vi "Tab Control Password 2012 NIVerified.vi"() -> ()   [LabVIEW 2020]
doc: "This is an example of how to password protect a tab control, which would be useful if an administrator wanted to restrict access to particular controls."
panel:
  in  "User (user)":string
  in  "OK Button":bool
  in  "Password (password)":string
  in  "stop":bool
  in  "Tab Control":T1(tab)
  out "User Name":string
  # "Overview: This is an example of how to password protect a tab control, which would be useful if an administrator wanted \nto restrict access to particular controls. \nRequirements: LabVIEW 2012 (or compatible)\nInstructions:\n1. Run the VI.\n2. Input the correct Password and User(the initial values are password and user, can be changed in Block Diagram) and click Enter.\n3. If the password and user are correct, the Password Protected Tab page will be enabled and display the user.\n4. If the password and/or user is incorrect, it will pop up a prompt dialog and stop the VI."
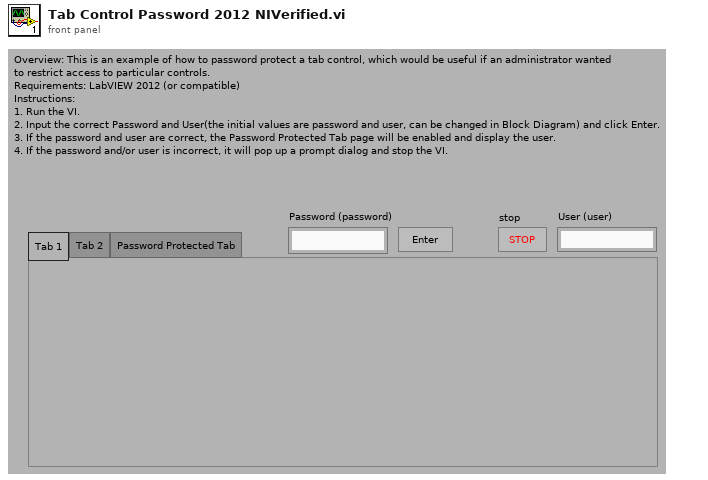
[diagram p1: front panel]
types:
  T1 = enum32{"Tab 1", "Tab 2", "Password Protected Tab"}
  T2 = enum32{"Page Enabled", "Page Disabled", "Page Disabled & Grayed"}
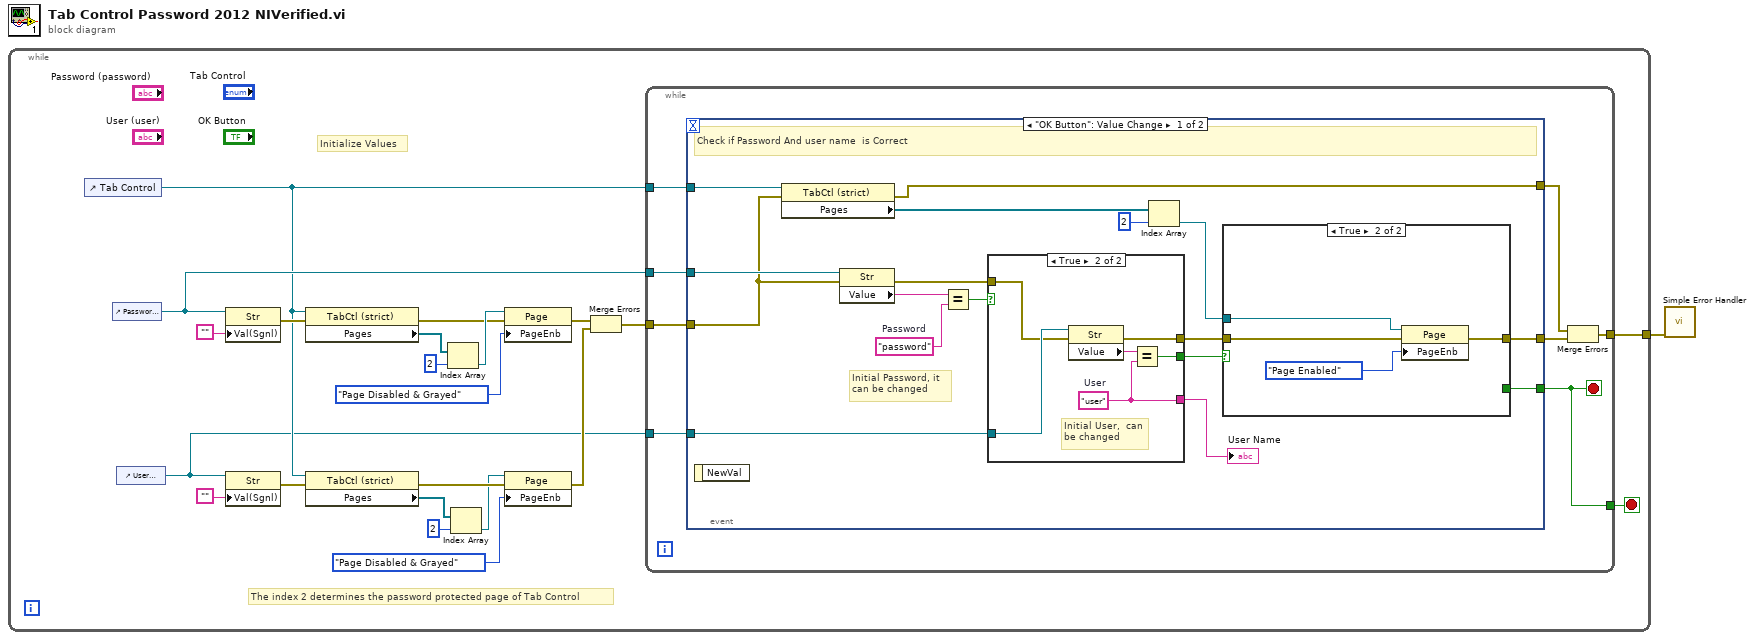
[diagram p0: block diagram]
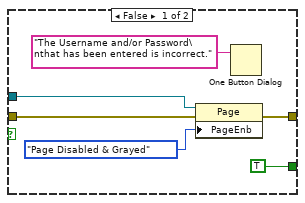
[diagram p2: hidden frame]
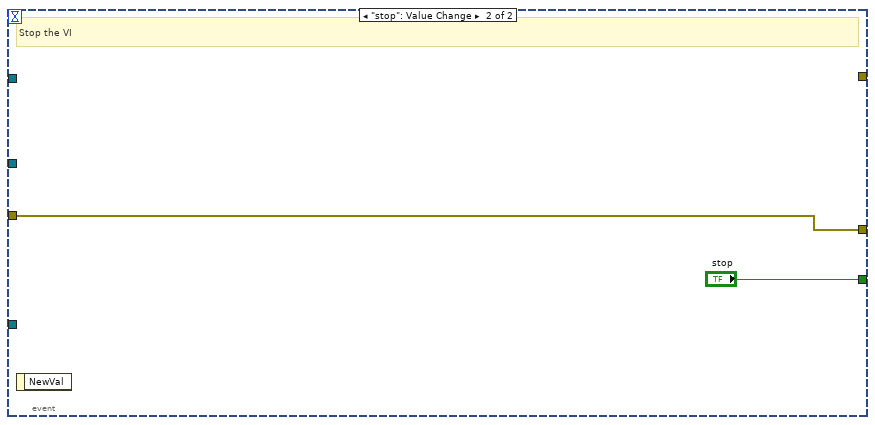
[diagram p4: hidden frame]
diagram:
  n1 = while {
    tunnel: [w2] -> w1
    stop <- w3 stop-if-true
    # "The index 2 determines the password protected page of Tab Control"
    # "Initialize Values"
    n2 = control-ref of="Tab Control"() -> (w5:refnum<vi>)
    n3 = control-ref of="Password (password)"() -> (w16:refnum<vi>)
    n4 = control-ref of="User (user)"() -> (w4:refnum<vi>)
    n5 = property on="Property Node" class="Str"(reference=w16, "Val(Sgnl)"="" ("Value (Signaling)")) -> (error out=w18:errorcluster)  [unwired: 1 in, 1 out]
    n6 = property on="Property Node" class="Str"(reference=w4, "Val(Sgnl)"="" ("Value (Signaling)")) -> (error out=w14:errorcluster)  [unwired: 1 in, 1 out]
    n7 = property on="Property Node" class="TabCtl (strict)"(reference=w5, error in=w18) -> (error out=w17:errorcluster, "Pages"=w20:refnum<vi>[])  [unwired: 1 out]
    n8 = property on="Property Node" class="TabCtl (strict)"(reference=w5, error in=w14) -> (error out=w13:errorcluster, "Pages"=w15:refnum<vi>[])  [unwired: 1 out]
    n9 = Index Array(array=w20, index=2) -> (element=w21:refnum<vi>)
    n10 = Index Array(array=w15, index=2) -> (element=w7:refnum<vi>)
    n11 = property on="Property Node" class="Page"(reference=w21, error in=w17, "PageEnb"=T2."Page Disabled & Grayed" ("Page Enabled State")) -> (error out=w9:errorcluster)  [unwired: 1 out]
    n12 = property on="Property Node" class="Page"(reference=w7, error in=w13, "PageEnb"=T2."Page Disabled & Grayed" ("Page Enabled State")) -> (error out=w10:errorcluster)  [unwired: 1 out]
    n13 = Merge Errors(w9, w10) -> (w8:errorcluster)
    n14 = while {
      tunnel: w5 -> [w31]
      tunnel: w8 -> [w30]
      tunnel: w16 -> [w29]
      tunnel: w4 -> [w28]
      tunnel: [w27] -> w3
      tunnel: [w24] -> w2
      stop <- w27 stop-if-true
      n15 = event shown="[0] \"OK Button\": Value Change" {
        selector: _ -> [_ _]
        dyn-events: _ -> [_ _]
        timeout: _ -> [_ _]
        tunnel: [w37 "stop"] -> w27
        tunnel: w31 -> [w45 _]
        tunnel: w30 -> [w36 w67]
        tunnel: w29 -> [w44 _]
        tunnel: w28 -> [w41 _]
        tunnel: [w33 w67] -> w25
        tunnel: [w32 _] -> w26
        event "OK Button": Value Change {
          w48 = "password"  # Password
          # "Initial Password, it \ncan be changed"
          # "Check if Password And user name  is Correct"
          n16 = event-data() -> ()  [unwired: 1 in, 1 out]
          n17 = property on="Property Node" class="TabCtl (strict)"(reference=w45, error in=w36) -> (error out=w32:errorcluster, "Pages"=w47:refnum<vi>[])  [unwired: 1 out]
          n18 = property on="Property Node" class="Str"(reference=w44, error in=w36) -> (error out=w35:errorcluster, "Value"=w43:string)  [unwired: 1 out]
          n19 = Equal?(x=w43, y=w48) -> (x = y?=w42:bool)
          n20 = case shown="True" w42 {
            selector: w42 -> [w60 _]
            tunnel: [w60 w65] -> w40
            tunnel: w41 -> [_ w64]
            tunnel: [_ w63] -> w38
            tunnel: w35 -> [w59 w62]
            tunnel: [w59 w61] -> w34
            frame False {
            }
            frame True {
              w63 = "user"  # User
              # "Initial User,  can\nbe changed"
              n21 = property on="Property Node" class="Str"(reference=w64, error in=w62) -> (error out=w61:errorcluster, "Value"=w66:string)  [unwired: 1 out]
              n22 = Equal?(x=w66, y=w63) -> (x = y?=w65:bool)
            }
          }
          "User Name" <- w38
          n23 = Index Array(array=w47, index=2) -> (element=w39:refnum<vi>)
          n24 = case shown="True" w40 {
            tunnel: w39 -> [w52 w57]
            tunnel: [TRUE ("stop") _] -> w37
            tunnel: w34 -> [w50 w56]
            tunnel: [w49 w55] -> w33
            frame False {
              n25 = property on="Property Node" class="Page"(reference=w52, error in=w50, "PageEnb"=T2."Page Disabled & Grayed" ("Page Enabled State")) -> (error out=w49:errorcluster)  [unwired: 1 out]
              n26 = One Button Dialog(message="The Username and/or Password\nthat has been entered is incorrect.") -> ()  [unwired: 1 in, 1 out]
            }
            frame True {
              n27 = property on="Property Node" class="Page"(reference=w57, error in=w56, "PageEnb"=T2."Page Enabled" ("Page Enabled State")) -> (error out=w55:errorcluster)  [unwired: 1 out]
            }
          }
        }
        event "stop": Value Change {
          # "Stop the VI"
          n28 = event-data() -> ()  [unwired: 1 in, 1 out]
        }
      }
      n29 = Merge Errors(w26, w25) -> (w24:errorcluster)
    }
  }
  n30 = call <vilib>:"Simple Error Handler.vi"("error in (no error)"=w1) -> ()  [unwired: 4 in, 5 out]
